vi "Binary to ASCII - Folder Version.vi"(8 "error in":errorcluster, 11 "file path (use dialog)":path) -> ()   [LabVIEW 2012]
uses:
  <vilib>/Utility/file.llb/Write To Spreadsheet File (DBL).vi
panel:
  out "appended path 2":path
  out "appended path":path
  out "error out 2":errorcluster
  out "filenames":string[](array[string])
  out "Waveform Graph":dbl[][](graph)
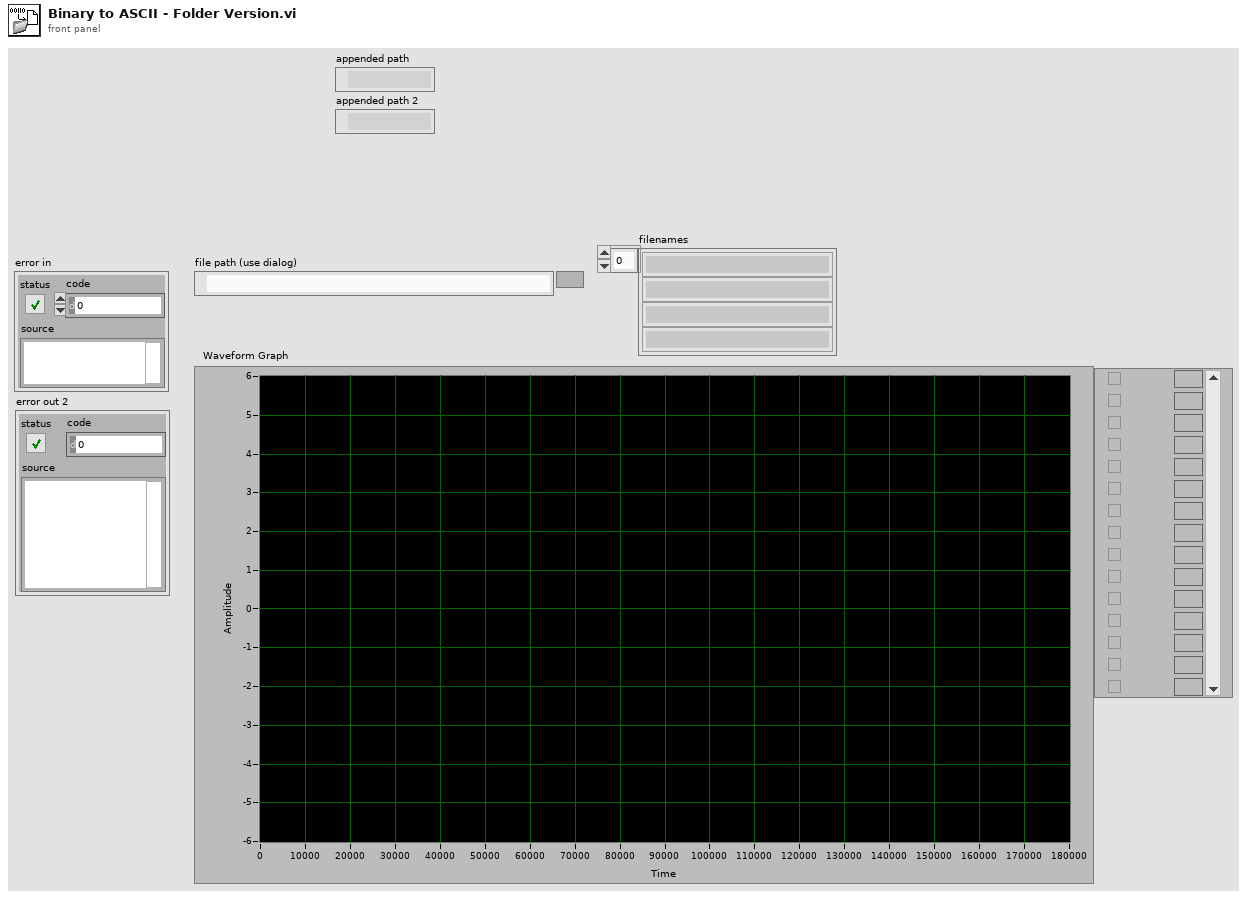
[diagram p1: front panel]
types:
  T1 = enum16{"open", "replace", "create", "open or create", "replace or create", "replace or create with confirmation"}
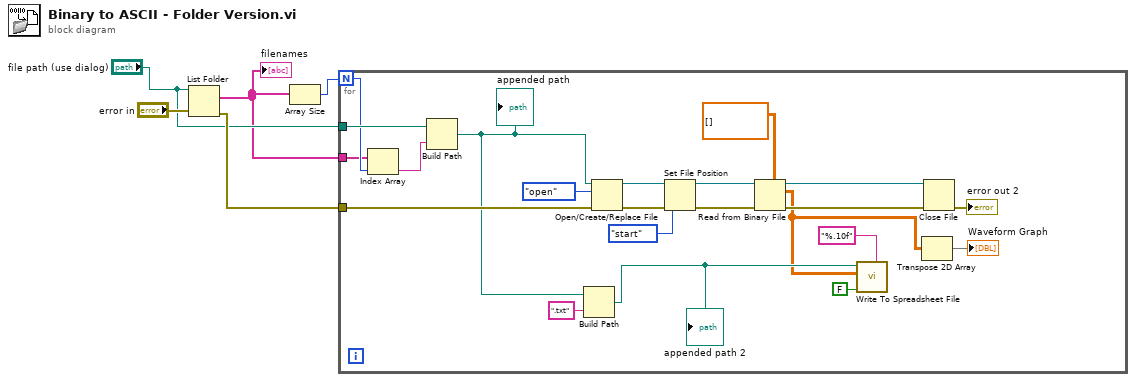
[diagram p0: block diagram]
diagram:
  n1 = List Folder(path="file path (use dialog)", error in="error in") -> (filenames=w2:string[], error out=w4:errorcluster)  [unwired: 2 in, 2 out]
  "filenames" <- w2
  n2 = Array Size(array=w2) -> (size(s)=w1:i32)
  n3 = for {
    N: w1 -> [w9]
    tunnel: w4 -> [w21]
    tunnel: "file path (use dialog)" -> [w10]
    tunnel: w2 -> [w8]
    n4 = Index Array(array=w8, index=w9) -> (element=w7:string)
    n5 = Build Path(base path=w10, name or relative path=w7) -> (appended path=w6:path)
    "appended path" <- w6
    n6 = Build Path(base path=w6, name or relative path=".txt") -> (appended path=w16:path)
    "appended path 2" <- w16
    n7 = Open/Create/Replace File(file path (use dialog)=w6, error in=w21, operation (0:open)=T1."open") -> (refnum out=w25:refnum<file>, error out=w23:errorcluster)  [unwired: 3 in, 1 out]
    n8 = Set File Position(refnum=w25, from (0:start)=enum16{"start", "end", "current"}."start", error in=w23) -> (refnum out=w26:refnum<file>, error out=w24:errorcluster)  [unwired: 1 in]
    n9 = Read from Binary File(5:dbl[][] [], 8:w24, 11:w26) -> (0:w13:errorcluster, 2:w12:dbl[][], 3:w14:refnum<file>)  [unwired: 3 in, 1 out]
    n10 = call-poly <vilib>:"Write To Spreadsheet File.vi"("format (%.3f)"="%.10f", "append to file? (new file:F)"=FALSE, "2D data"=w12, "file path (dialog if empty)"=w16) -> ()  [unwired: 4 in, 1 out]
    n11 = Transpose 2D Array(2D array=w12) -> (transposed array=→"Waveform Graph":dbl[][])
    n12 = Close File(refnum=w14, error in=w13) -> (error out=→"error out 2":errorcluster)  [unwired: 1 out]
  }
